vi "Cache-Broadcast Registry Search Result.vi"(8 "error in (no error)":errorcluster, 10 "CSM Name":string, 11 "Broadcast state":string) -> (0 "error out":errorcluster, 3 "Array":T2(array[cluster]))   [LabVIEW 2020, in "Communicable State Machine.lvlib"]
uses:
  Communicable State Machine.lvlib
  CSM - Broadcast Message Type.ctl
  _CSMOFGVOPER.ctl
  Operation-BroadcastRegistry.ctl
  global-CSMQ FGV Change Flag.vi
  global-Broadcast Cache Change Flag.vi
  BroadcastRegistry.lvclass
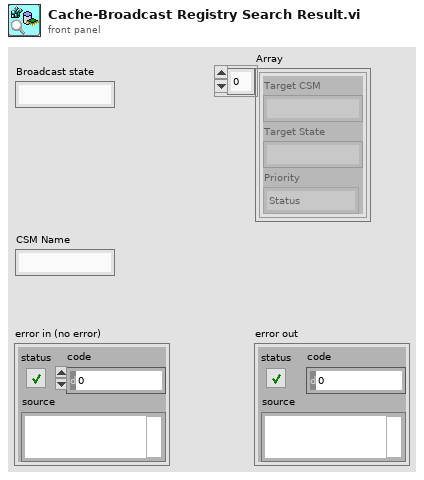
[diagram p1: front panel]
types:
  T1 = typedef "Communicable State Machine.lvlib/CSM - Broadcast Message Type.ctl" = enum16{"Status", "Interrupt(High)"}
  T2 = cluster{"Target CSM":string, "Target State":string, "Priority":T1}[]
  T3 = cluster{"Target CSM":string, "Target State":string, "Priority":T1}
  T4 = typedef "Communicable State Machine.lvlib/_CSMOFGVOPER.ctl" = enum16{"Create If not Exist", "Get By Name", "List", "Check If Name Exists", "Release", "Module Status", "Create Status Event Handler", "Destroy Status Event Handler"}
  T5 = typedef "Communicable State Machine.lvlib/Operation-BroadcastRegistry.ctl" = enum16{"Delete Source Module", "Delete Target Module", "Remove Module", "Register", "Unregister", "Check", "List Status", "List Entries"}
  T6 = typedef "Communicable State Machine.lvlib/_CSMObj.ctl" = cluster{"Requested Name":string, "Module Name":string, "Mode":T7, "Queue":refnum<class "Priority Queue.lvclass">, "CSM-Data":refnum<data-value>, "User Event":refnum<user-event>, "Status Change Event":refnum<user-event>, "Allowed Messages":string[], "Mode-Data":refnum<data-value>, "Group Name":string, "Exit Event":refnum<user-event>}
  T7 = typedef "Communicable State Machine.lvlib/_CSM_MODE.ctl" = enum16{"Not Exist", "Stand Alone", "CSM", "Worker Agent", "Worker", "Chain", "Chain Node"}
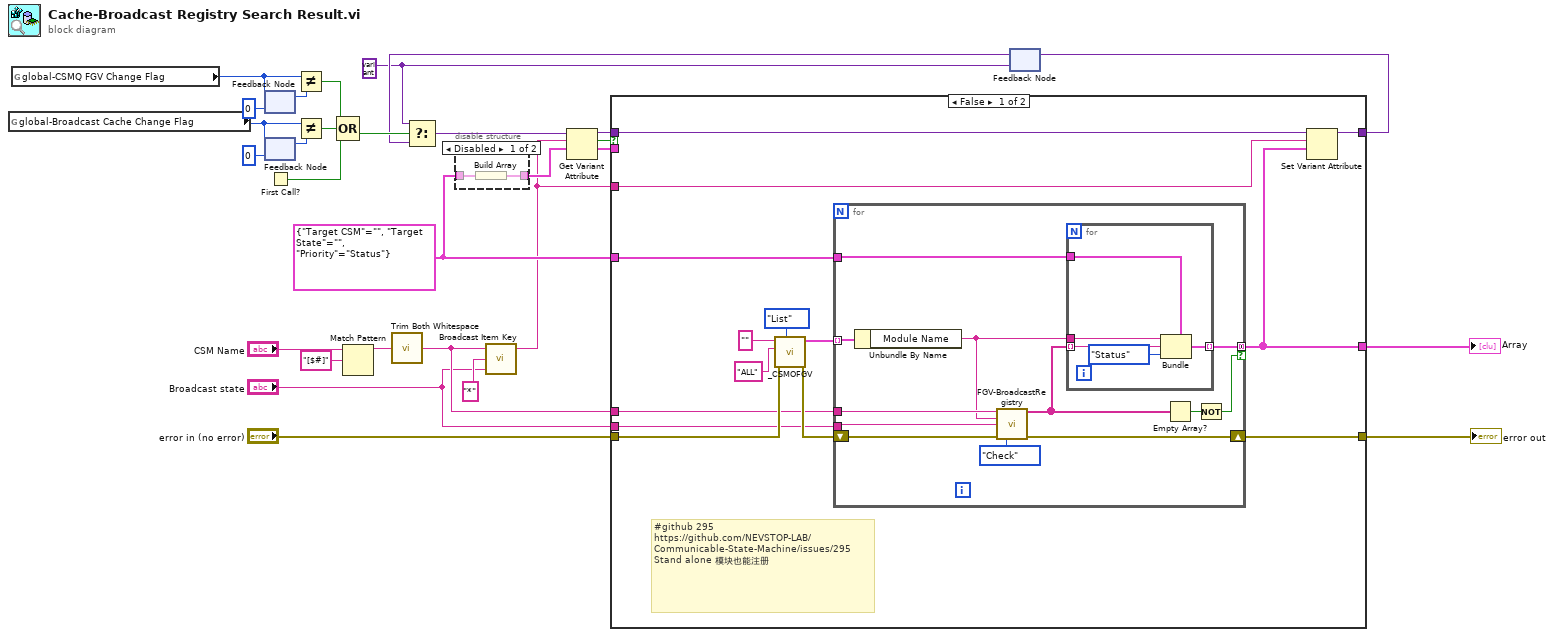
[diagram p0: block diagram]
diagram:
  w20 = T3 {"Target CSM"="", "Target State"="", "Priority"=enum."Status"} ("cluster")
  w22 = variant
  n1 = global read "global-Broadcast Cache Change Flag.vi" "global-Broadcast Cache Change Flag"() -> (w14:u64)
  n2 = global read "global-CSMQ FGV Change Flag.vi" "global-CSMQ FGV Change Flag"() -> (w6:u64)
  n3 = feedback #1(u64 0 ("global-Broadcast Cache Change Flag")) -> (w7:u64)
  n4 = feedback-in #1(w6) -> ()
  n5 = feedback #2(u64 0 ("global-Broadcast Cache Change Flag")) -> (w13:u64)
  n6 = feedback-in #2(w14) -> ()
  n7 = First Call?() -> (First Call?: T/F=w25:bool)
  n8 = Not Equal?(x=w6, y=w7) -> (x != y?=w5:bool)
  n9 = Not Equal?(x=w14, y=w13) -> (x != y?=w26:bool)
  n10 = Compound Arithmetic op=OR(w5, w26, w25) -> (w24:bool)
  n11 = Match Pattern(string="CSM Name", regular expression="[$#]") -> (before substring=w11:string)  [unwired: 1 in, 3 out]
  n12 = call "Trim Both Whitespace.vi"("string"=w11) -> ("trimmed string"=w4:string)  [unwired: 1 in]
  n13 = disable-structure shown="Disabled" {
    disable-tunnel: w20 -> [w31 _]
    disable-tunnel: [w30 _] -> w19
    frame Disabled {
      n14 = Build Array(w31) -> (w30:T2)
    }
    frame Enabled {
    }
  }
  n15 = call "Broadcast Item Key.vi"("status"="Broadcast state", "target"="*", "source"=w4) -> ("key"=w1:string)  [unwired: 2 in]
  n16 = feedback #3(w22) -> (w23:variant)
  n17 = Select(t=w22, s=w24, f=w23) -> (s? t:f=w21:variant)
  n18 = Get Variant Attribute(Variant=w21, name=w1, default value (empty Variant)=w19) -> (duplicate Variant=w17:variant, found=w18:bool, value=w16:T2)  [unwired: 1 in, 1 out]
  n19 = case shown="False" w18 {
    tunnel: [w45 w64] -> w29
    tunnel: "error in (no error)" -> [w43 w64]
    tunnel: [w36 w65] -> w27
    tunnel: "Broadcast state" -> [w41 _]
    tunnel: w4 -> [w40 _]
    tunnel: w20 -> [w39 _]
    tunnel: w17 -> [w38 w63]
    tunnel: w16 -> [_ w65]
    tunnel: w1 -> [w37 _]
    tunnel: [w35 w63] -> w15
    frame False {
      # "#github 295\nhttps://github.com/NEVSTOP-LAB/Communicable-State-Machine/issues/295\nStand alone 模块也能注册"
      n20 = call "_CSMOFGV.vi"("Operation"=_CSMOFGVOPER."List", "Error in"=w43, "Reference"="ALL" ("Name(\"\" to use uuid) in"), "Name(\"\" to use uuid) in"="" ("Name(\"\" to use uuid) in")) -> ("Error out"=w44:errorcluster, "Array"=w34:T6[])  [unwired: 5 in, 1 out]
      n21 = for {
        tunnel: w34 -> [w53] mode=indexing
        tunnel: w40 -> [w55]
        tunnel: w41 -> [w51]
        shift-right: [w54] -> w45
        shift-left: w44 -> [w56]
        tunnel: [w50] -> w36 mode=concatenating if=w52
        tunnel: w39 -> [w49]
        n22 = Unbundle By Name(w53) -> ("Module Name"=w48:string)
        n23 = call "FGV-BroadcastRegistry.vi"("Source"=w55, "Target"=w48, "Status"=w51, "Error in"=w56, "Operation"=Operation-BroadcastRegistry."Check") -> ("response message"=w46:string[], "Error out"=w54:errorcluster)  [unwired: 9 in]
        n24 = for {
          tunnel: w48 -> [w60]
          tunnel: w49 -> [w61]
          tunnel: [w62] -> w50 mode=indexing
          tunnel: w46 -> [w59] mode=indexing
          n25 = Bundle(cluster=w61, "Target CSM"=w60, "Target State"=w59, "Priority"=CSM_-_Broadcast_Message_Type."Status") -> (w62:T3)
        }
        n26 = Empty Array?(array=w46) -> (empty?=w47:bool)
        n27 = Not(x=w47) -> (.not. x?=w52:bool)
      }
      n28 = Set Variant Attribute(Variant=w38, name=w37, value=w36) -> (Variant out=w35:variant)  [unwired: 1 in, 2 out]
    }
    frame True {
    }
  }
  "error out" <- w29
  "Array" <- w27
  n29 = feedback-in #3(w15) -> ()
